vi "Next Frame.vi"(8 "error in (no error)":errorcluster, 11 "[V] Main UI in":refnum<class "[V] Main UI.lvclass">) -> (0 "error out":errorcluster, 3 "[V] Main UI out":refnum<class "[V] Main UI.lvclass">)   [LabVIEW 2020, in "[V] Main UI.lvlib" / "[V] Main UI.lvclass"]
uses:
  [V] Main UI.lvclass
  [V] Main UI.lvclass/[V] Main UI.ctl
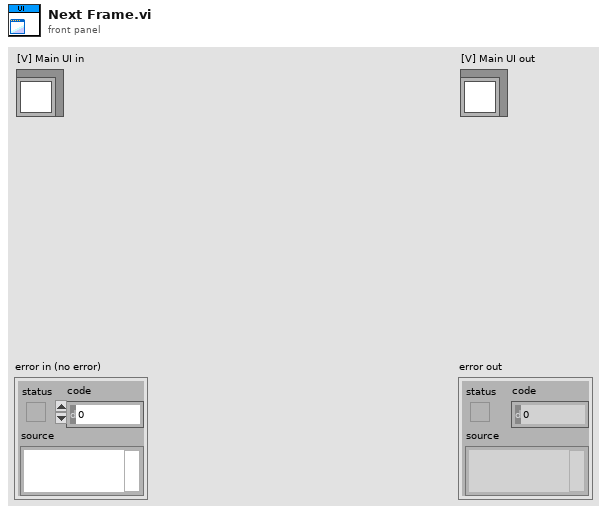
[diagram p1: front panel]
types:
  T1 = typedef "number.ctl" = i8
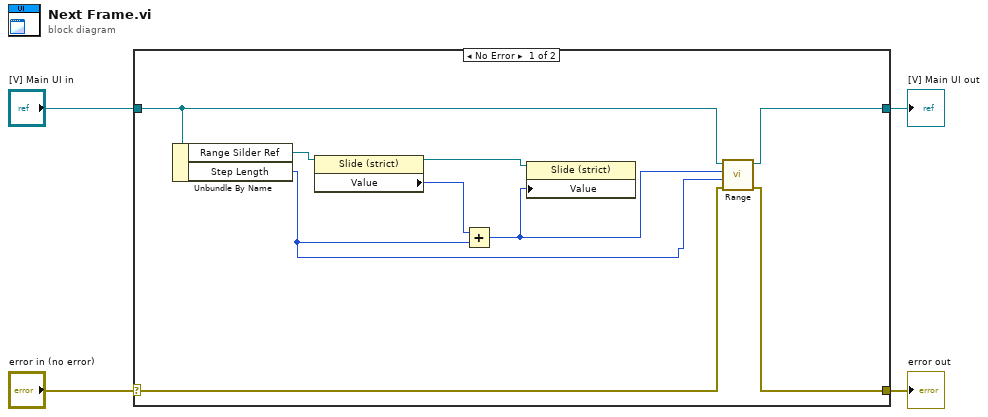
[diagram p0: block diagram]
diagram:
  n1 = case shown="No Error" "error in (no error)" {
    selector: "error in (no error)" -> [w9 w15]
    tunnel: [w8 w15] -> w3
    tunnel: [w10 w14] -> w1
    tunnel: "[V] Main UI in" -> [w11 w14]
    frame No Error {
      n2 = Unbundle By Name(w11) -> ("Range Silder Ref"=w13:refnum<vi>, "Step Length"=w5:u8)
      n3 = property class="Slide (strict)"(reference=w13) -> (reference out=w7:refnum<vi>, "Value"=w12:T1)  [unwired: 1 in, 1 out]
      n4 = Add(x=w12, y=w5) -> (x+y=w6:u8)
      n5 = property class="Slide (strict)"(reference=w7, "Value"=w6) -> ()  [unwired: 1 in, 2 out]
      n6 = call "Range.vi"("error in (no error)"=w9, "length"=w5, "index"=w6, "[V] Main UI in"=w11) -> ("error out"=w8:errorcluster, "[V] Main UI out"=w10:refnum<class "[V] Main UI.lvclass">)  [unwired: 6 in]
    }
    frame Error {
    }
  }
  "error out" <- w3
  "[V] Main UI out" <- w1
